vi "ParseConfCases.vi"(11 "DataIn":string[][](array[string])) -> (1 "StateData":T1(array[cluster]), 2 "CountyData":T2(array[cluster]), 3 "Days":timestamp[](array[timestamp]))   [LabVIEW 2017]
uses:
  <vilib>/Utility/miscctls.llb/LVDateTimeRec.ctl
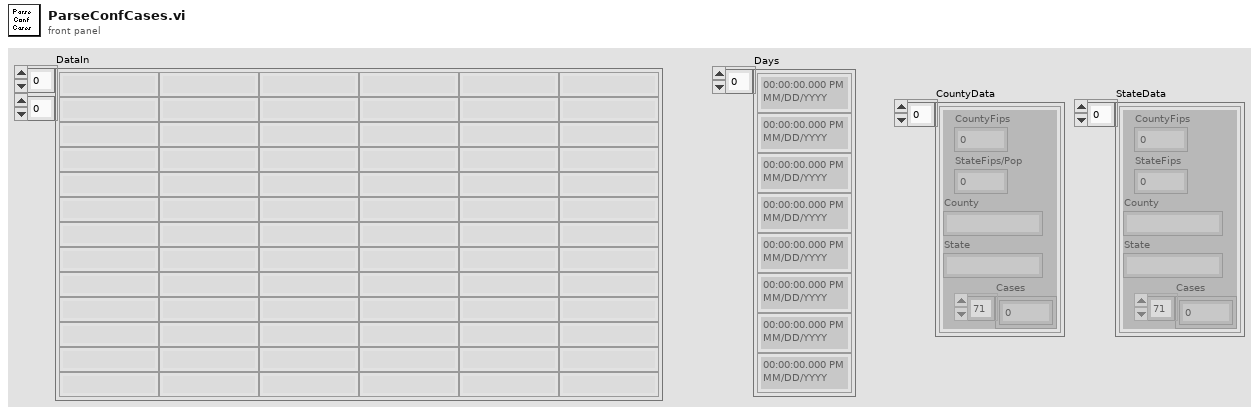
[diagram p1: front panel]
types:
  T1 = cluster{"CountyFips":i32, "StateFips":i32, "County":string, "State":string, "Cases":i32[]}[]
  T2 = cluster{"CountyFips":i32, "StateFips/Pop":i32, "County":string, "State":string, "Cases":i32[]}[]
  T3 = typedef "LVDateTimeRec.ctl" = cluster{"fractional second":dbl, "second":i32, "minute":i32, "hour":i32, "day of month":i32, "month":i32, "year":i32, "day of week":i32, "day of year":i32, "DST":i32}
  T4 = cluster{"CountyFips":i32, "StateFips":i32, "County":string, "State":string, "Cases":i32[]}
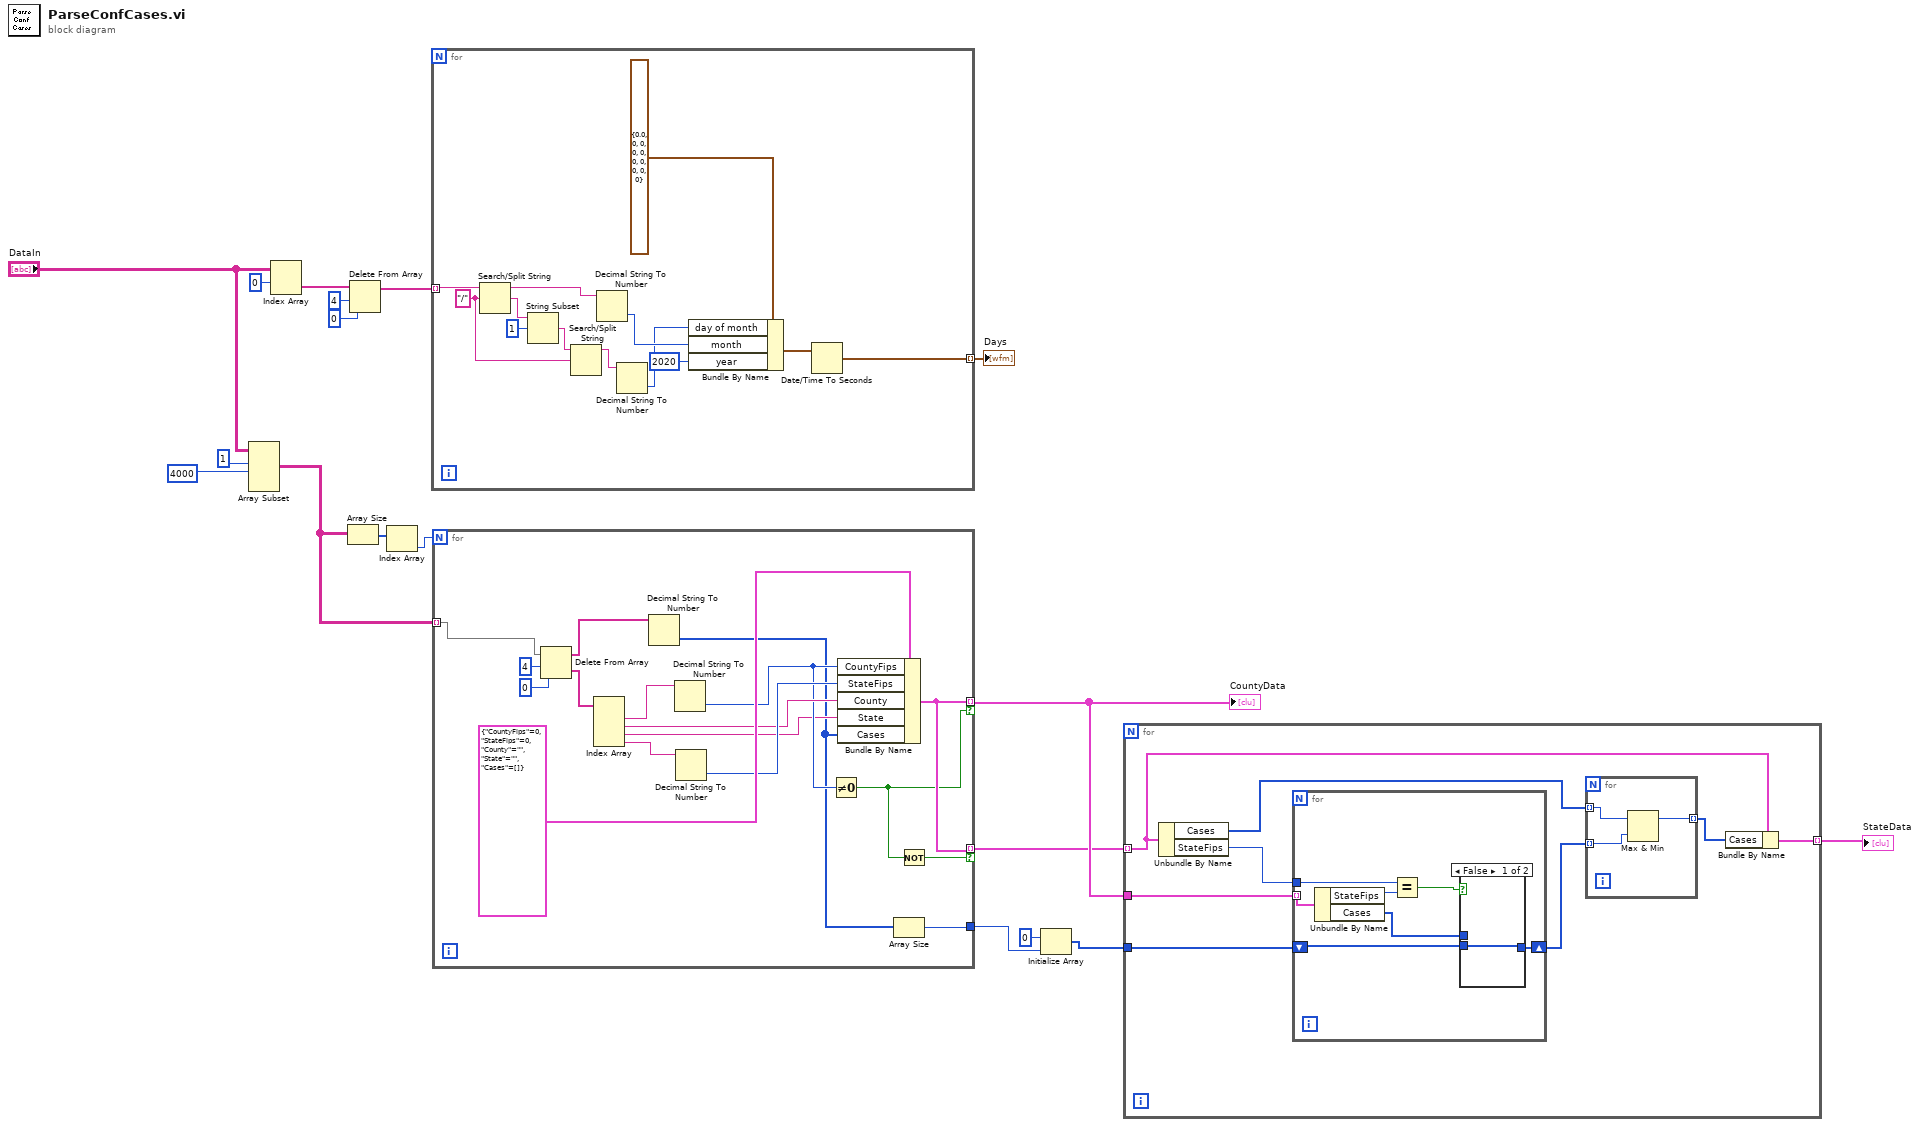
[diagram p0: block diagram]
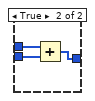
[diagram p2: hidden frame]
diagram:
  n1 = Array Subset(array="DataIn", index (row)=1 ("index"), length (row)=4000 ("length")) -> (w9:string[][])  [unwired: 2 in]
  n2 = Index Array(array="DataIn", index (row)=0) -> (element=w17:string[])  [unwired: 1 in]
  n3 = Array Size(array=w9) -> (size(s)=w8:i32[])
  n4 = Delete From Array(array=w17, length=4, index=0) -> (array with subset deleted=w15:string[])  [unwired: 1 out]
  n5 = Index Array(array=w8) -> (element=w7:i32)  [unwired: 1 in]
  n6 = for {
    tunnel: w15 -> [w30] mode=indexing
    tunnel: [w23] -> w14 mode=indexing
    w27 = "/" ("search string/char (-)")
    n7 = Search/Split String(string=w30, search string/char (-)=w27) -> (substring before match=w29:string, match + rest of string=w22:string)  [unwired: 1 in, 1 out]
    n8 = String Subset(string=w22, offset (0)=1) -> (substring=w20:string)  [unwired: 1 in]
    n9 = Search/Split String(string=w20, search string/char (-)=w27) -> (substring before match=w26:string)  [unwired: 1 in, 2 out]
    n10 = Decimal String To Number(string=w29) -> (number=w28:i32)  [unwired: 2 in, 1 out]
    n11 = Decimal String To Number(string=w26) -> (number=w25:i32)  [unwired: 2 in, 1 out]
    n12 = Bundle By Name(cluster=T3 {"fractional second"=0.0, "second"=0, "minute"=0, "hour"=0, "day of month"=0, "month"=0, "year"=0, "day of week"=0, "day of year"=0, "DST"=0} ("date time rec"), "day of month"=w25, "month"=w28, "year"=2020) -> (w24:T3)
    n13 = Date/Time To Seconds(2:w24) -> (0:w23:timestamp)  [unwired: 1 in]
  }
  "Days" <- w14
  n14 = for {
    N: w7 -> [_]
    tunnel: w9 -> [w40] mode=indexing
    tunnel: [w36] -> w6 mode=indexing if=w35
    tunnel: [w36] -> w4 mode=indexing if=w34
    tunnel: [w32] -> w3
    n15 = Delete From Array(array=w40, length=4, index=0) -> (deleted portion=w46:string[], array with subset deleted=w47:string[])
    n16 = Index Array(array=w46) -> (element #1=w45:string, element #2=w42:string, element #3=w37:string, element #4=w38:string)  [unwired: 4 in]
    n17 = Decimal String To Number(string=w47) -> (number=w33:i32[])  [unwired: 2 in, 1 out]
    n18 = Decimal String To Number(string=w45) -> (number=w41:i32)  [unwired: 2 in, 1 out]
    n19 = Decimal String To Number(string=w38) -> (number=w43:i32)  [unwired: 2 in, 1 out]
    n20 = Not Equal To 0?(x=w41) -> (x != 0?=w35:bool)
    n21 = Bundle By Name(cluster=T4 {"CountyFips"=0, "StateFips"=0, "County"="", "State"="", "Cases"=[]}, "CountyFips"=w41, "StateFips"=w43, "County"=w42, "State"=w37, "Cases"=w33) -> (w36:T4)
    n22 = Array Size(array=w33) -> (size(s)=w32:i32)
    n23 = Not(x=w35) -> (.not. x?=w34:bool)
  }
  "CountyData" <- w6
  n24 = Initialize Array(0 ("element"), w3) -> (w1:i32[])
  n25 = for {
    tunnel: w4 -> [w51] mode=indexing
    tunnel: w6 -> [w56]
    tunnel: w1 -> [w54]
    tunnel: [w49] -> w5 mode=indexing
    n26 = Unbundle By Name(w51) -> ("Cases"=w53:i32[], "StateFips"=w55:i32)
    n27 = for {
      tunnel: w56 -> [w66] mode=indexing
      tunnel: w55 -> [w64]
      shift-right: [w63] -> w52
      shift-left: w54 -> [w61]
      n28 = Unbundle By Name(w66) -> ("StateFips"=w65:i32, "Cases"=w62:i32[])
      n29 = Equal?(x=w64, y=w65) -> (x = y?=w60:bool)
      n30 = case shown="False" w60 {
        tunnel: [w67 w70] -> w63
        tunnel: w62 -> [_ w69]
        tunnel: w61 -> [w67 w68]
        frame False {
        }
        frame True {
          n31 = Add(x=w69, y=w68) -> (x+y=w70:i32[])
        }
      }
    }
    n32 = for {
      tunnel: w53 -> [w59] mode=indexing
      tunnel: w52 -> [w58] mode=indexing
      tunnel: [w57] -> w50 mode=indexing
      n33 = Max & Min(x=w59, y=w58) -> (max(x,y)=w57:i32)  [unwired: 1 out]
    }
    n34 = Bundle By Name(cluster=w51, "Cases"=w50) -> (w49:T4)
  }
  "StateData" <- w5
